vi "数据索引起始时间填补空白.vi"(8 "error in (no error)":errorcluster caption="错误输入（无错误）") -> (0 "error out":errorcluster caption="错误输出")   [LabVIEW 2016, in "数据传输系统.lvlib"]
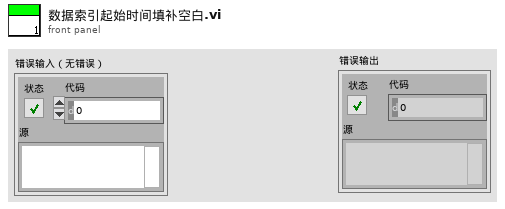
[diagram p1: front panel]
types:
  T1 = typedef "LVDateTimeRec.ctl" = cluster{"秒数的小数部分":dbl, "秒":i32, "分":i32, "时":i32, "日":i32, "月":i32, "年":i32, "天数（周）":i32, "天数（年）":i32, "DST":i32}
  T2 = cluster{"氨氮仪器参数索引起始时间":string, "总磷仪器参数索引起始时间":string, "总氮仪器参数索引起始时间":string, "CODMn仪器参数索引起始时间":string, "CODCr仪器参数索引起始时间":string, "DO仪器参数索引起始时间":string, "PH仪器参数索引起始时间":string, "比电导率仪器参数索引起始时间":string, "水温仪器参数索引起始时间":string, "浊度仪器参数索引起始时间":string, "叶绿素a仪器参数索引起始时间":string, "藻密度仪器参数索引起始时间":string, "ORP仪器参数索引起始时间":string}
  T3 = cluster{"氨氮加标回收索引起始时间":string, "总磷加标回收索引起始时间":string, "总氮加标回收索引起始时间":string, "CODMn加标回收索引起始时间":string, "CODCr加标回收索引起始时间":string}
  T4 = cluster{"氨氮标样核查索引起始时间":string, "总磷标样核查索引起始时间":string, "总氮标样核查索引起始时间":string, "CODMn标样核查索引起始时间":string, "CODCr标样核查索引起始时间":string, "DO标样核查索引起始时间":string, "PH标样核查索引起始时间":string, "比电导率标样核查索引起始时间":string, "水温标样核查索引起始时间":string, "浊度标样核查索引起始时间":string, "叶绿素a标样核查索引起始时间":string, "藻密度标样核查索引起始时间":string, "亚硝酸盐标样核查索引起始时间":string, "硫化物标样核查索引起始时间":string, "ORP标样核查索引起始时间":string}
  T5 = cluster{"氨氮跨度核查索引起始时间":string, "总磷跨度核查索引起始时间":string, "总氮跨度核查索引起始时间":string, "CODMn跨度核查索引起始时间":string, "CODCr跨度核查索引起始时间":string, "亚硝酸盐跨度核查索引起始时间":string, "硫化物跨度核查索引起始时间":string, "ORP跨度核查索引起始时间":string}
  T6 = cluster{"氨氮报警信息索引起始时间":string, "总磷报警信息索引起始时间":string, "总氮报警信息索引起始时间":string, "CODMn报警信息索引起始时间":string, "CODCr报警信息索引起始时间":string, "DO报警信息索引起始时间":string, "PH报警信息索引起始时间":string, "比电导率报警信息索引起始时间":string, "水温报警信息索引起始时间":string, "浊度报警信息索引起始时间":string, "叶绿素报警信息索引起始时间":string, "系统报警信息索引起始时间":string}
  T7 = cluster{"氨氮集成干预索引起始时间":string, "总磷集成干预索引起始时间":string, "总氮集成干预索引起始时间":string, "CODMn集成干预索引起始时间":string, "CODCr集成干预索引起始时间":string, "DO集成干预索引起始时间":string, "PH集成干预索引起始时间":string, "比电导率集成干预索引起始时间":string, "水温集成干预索引起始时间":string, "浊度集成干预索引起始时间":string, "叶绿素a集成干预索引起始时间":string, "藻密度集成干预索引起始时间":string, "亚硝酸盐集成干预索引起始时间":string, "硫化物集成干预索引起始时间":string, "ORP集成干预索引起始时间":string}
  T8 = cluster{"氨氮仪器日志索引起始时间":string, "总磷仪器日志索引起始时间":string, "总氮仪器日志索引起始时间":string, "CODMn仪器日志索引起始时间":string, "CODCr仪器日志索引起始时间":string, "系统仪器日志索引起始时间":string}
  T9 = cluster{"氨氮零点核查索引起始时间":string, "总磷零点核查索引起始时间":string, "总氮零点核查索引起始时间":string, "CODMn零点核查索引起始时间":string, "CODCr零点核查索引起始时间":string, "亚硝酸盐零点核查索引起始时间":string, "硫化物零点核查索引起始时间":string, "ORP零点核查索引起始时间":string}
  T10 = cluster{"氨氮平行样索引起始时间":string, "总磷平行样索引起始时间":string, "总氮平行样索引起始时间":string, "CODMn平行样索引起始时间":string, "CODCr平行样索引起始时间":string}
  T11 = cluster{"[0]":string, "[1]":string, "[2]":string, "[3]":string, "[4]":string, "[5]":string, "[6]":string, "[7]":string, "[8]":string, "[9]":string, "[10]":string, "[11]":string, "[12]":string}
  T12 = cluster{"[0]":string, "[1]":string, "[2]":string, "[3]":string, "[4]":string}
  T13 = cluster{"[0]":string, "[1]":string, "[2]":string, "[3]":string, "[4]":string, "[5]":string, "[6]":string, "[7]":string, "[8]":string, "[9]":string, "[10]":string, "[11]":string, "[12]":string, "[13]":string, "[14]":string}
  T14 = cluster{"[0]":string, "[1]":string, "[2]":string, "[3]":string, "[4]":string, "[5]":string, "[6]":string, "[7]":string}
  T15 = cluster{"[0]":string, "[1]":string, "[2]":string, "[3]":string, "[4]":string, "[5]":string, "[6]":string, "[7]":string, "[8]":string, "[9]":string, "[10]":string, "[11]":string}
  T16 = cluster{"[0]":string, "[1]":string, "[2]":string, "[3]":string, "[4]":string, "[5]":string}
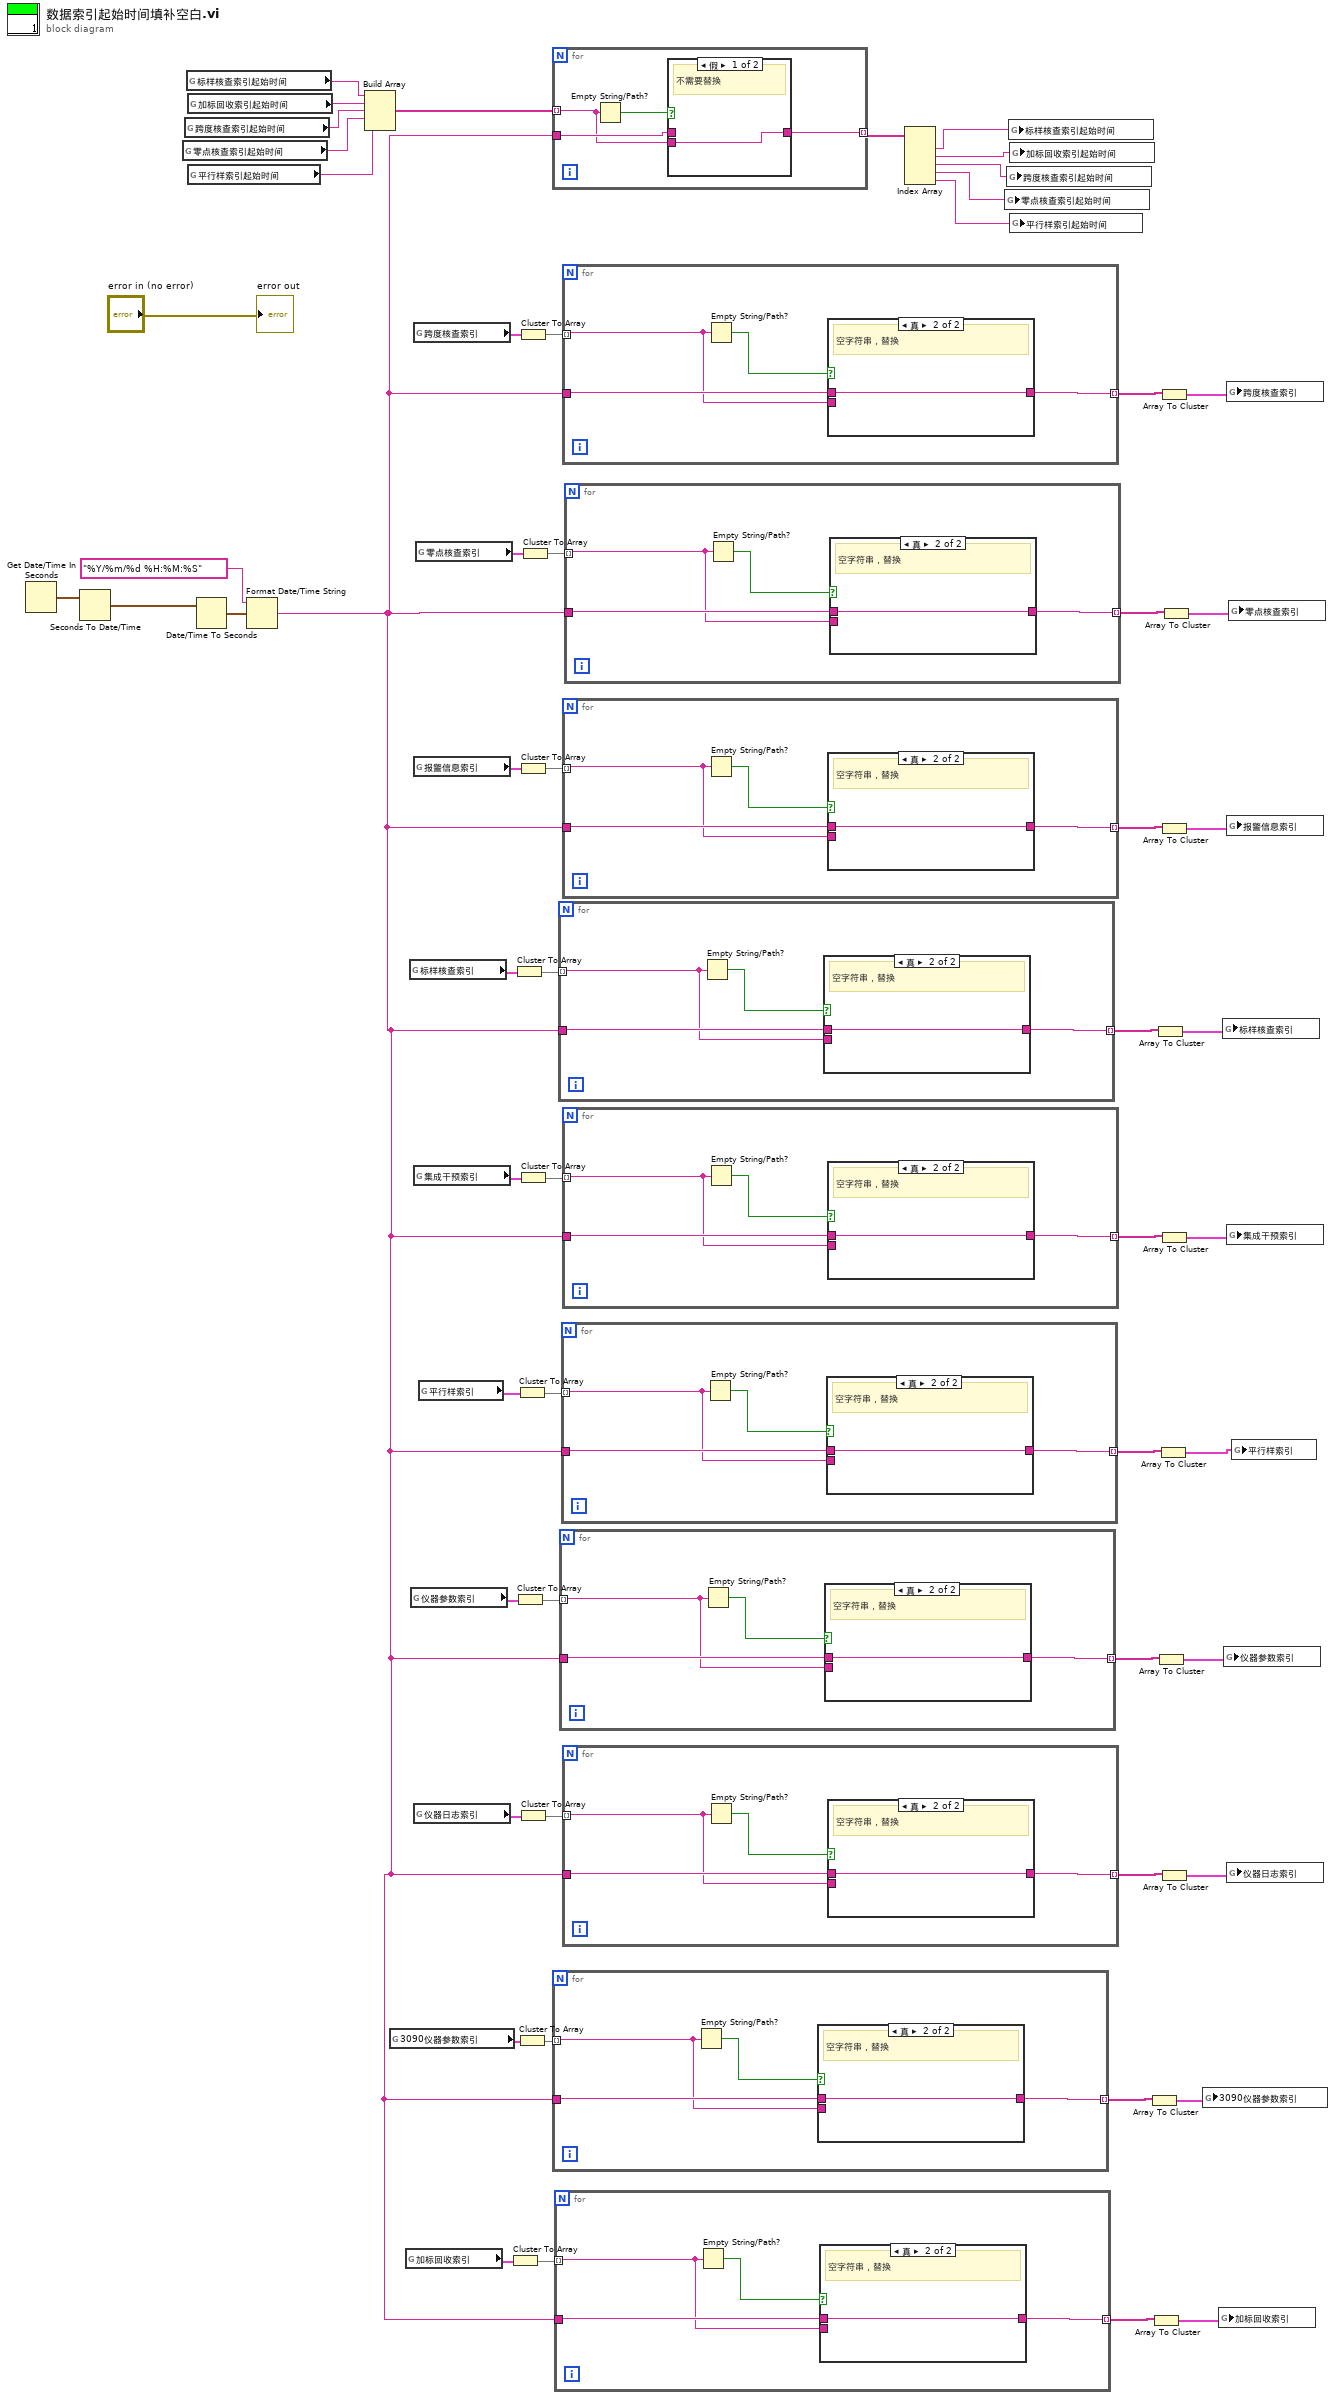
[diagram p0: block diagram]
diagram:
  n1 = Get Date/Time In Seconds() -> (seconds since 1Jan1904=w58:timestamp)
  n2 = Seconds To Date/Time(time stamp (now)=w58) -> (date time rec=w56:T1)  [unwired: 1 in]
  n3 = global read "全局 时间2.vi" "零点核查索引起始时间"() -> (w17:string)
  n4 = global read "全局 时间2.vi" "跨度核查索引起始时间"() -> (w19:string)
  n5 = global read "全局 时间2.vi" "标样核查索引起始时间"() -> (w21:string)
  n6 = global read "全局 时间2.vi" "加标回收索引起始时间"() -> (w20:string)
  n7 = global read "全局 时间2.vi" "平行样索引起始时间"() -> (w18:string)
  n8 = Date/Time To Seconds(2:w56) -> (0:w55:timestamp)  [unwired: 1 in]
  n9 = Format Date/Time String(time format string (%c)="%Y/%m/%d %H:%M:%S" ("时间格式字符串(%c)"), seconds (now)=w55) -> (date/time string=w1:string)  [unwired: 1 in]
  n10 = Build Array(w21, w20, w19, w17, w18) -> (w16:string[])
  n11 = global read "全局 时间2.vi" "3090仪器参数索引"() -> (w9:T2)
  n12 = global read "全局 时间2.vi" "加标回收索引"() -> (w5:T3)
  n13 = global read "全局 时间2.vi" "标样核查索引"() -> (w46:T4)
  n14 = global read "全局 时间2.vi" "仪器参数索引"() -> (w27:T2)
  n15 = global read "全局 时间2.vi" "跨度核查索引"() -> (w35:T5)
  n16 = global read "全局 时间2.vi" "报警信息索引"() -> (w47:T6)
  n17 = global read "全局 时间2.vi" "集成干预索引"() -> (w39:T7)
  n18 = global read "全局 时间2.vi" "仪器日志索引"() -> (w26:T8)
  n19 = global read "全局 时间2.vi" "零点核查索引"() -> (w54:T9)
  n20 = global read "全局 时间2.vi" "平行样索引"() -> (w34:T10)
  n21 = Cluster To Array(cluster=w5) -> (array=w4:string[])
  n22 = Cluster To Array(cluster=w46) -> (array=w45:string[])
  n23 = Cluster To Array(cluster=w27) -> (array=w28:string[])
  n24 = Cluster To Array(cluster=w34) -> (array=w33:string[])
  n25 = Cluster To Array(cluster=w9) -> (array=w8:string[])
  n26 = Cluster To Array(cluster=w35) -> (array=w36:string[])
  n27 = Cluster To Array(cluster=w47) -> (array=w48:string[])
  n28 = Cluster To Array(cluster=w39) -> (array=w40:string[])
  n29 = Cluster To Array(cluster=w26) -> (array=w25:string[])
  n30 = Cluster To Array(cluster=w54) -> (array=w53:string[])
  n31 = for {
    tunnel: w16 -> [w60] mode=indexing
    tunnel: w1 -> [w61]
    tunnel: [w59] -> w15 mode=indexing
    n32 = Empty String/Path?(string/path=w60) -> (empty?=w62:bool)
    n33 = case shown="假" w62 {
      tunnel: w61 -> [_ w64]
      tunnel: [w63 w64] -> w59
      tunnel: w60 -> [w63 _]
      frame False {
        # "不需要替换"
      }
      frame True {
        # "空字符串，替换"
      }
    }
  }
  n34 = for {
    tunnel: w8 -> [w65] mode=indexing
    tunnel: w1 -> [w67]
    tunnel: [w66] -> w7 mode=indexing
    n35 = Empty String/Path?(string/path=w65) -> (empty?=w68:bool)
    n36 = case shown="真" w68 {
      tunnel: w67 -> [_ w70]
      tunnel: [w69 w70] -> w66
      tunnel: w65 -> [w69 _]
      frame False {
        # "不需要替换"
      }
      frame True {
        # "空字符串，替换"
      }
    }
  }
  n37 = for {
    tunnel: w4 -> [w71] mode=indexing
    tunnel: w1 -> [w73]
    tunnel: [w72] -> w3 mode=indexing
    n38 = Empty String/Path?(string/path=w71) -> (empty?=w74:bool)
    n39 = case shown="真" w74 {
      tunnel: w73 -> [_ w76]
      tunnel: [w75 w76] -> w72
      tunnel: w71 -> [w75 _]
      frame False {
        # "不需要替换"
      }
      frame True {
        # "空字符串，替换"
      }
    }
  }
  n40 = for {
    tunnel: w45 -> [w77] mode=indexing
    tunnel: w1 -> [w79]
    tunnel: [w78] -> w44 mode=indexing
    n41 = Empty String/Path?(string/path=w77) -> (empty?=w80:bool)
    n42 = case shown="真" w80 {
      tunnel: w79 -> [_ w82]
      tunnel: [w81 w82] -> w78
      tunnel: w77 -> [w81 _]
      frame False {
        # "不需要替换"
      }
      frame True {
        # "空字符串，替换"
      }
    }
  }
  n43 = for {
    tunnel: w28 -> [w83] mode=indexing
    tunnel: w1 -> [w85]
    tunnel: [w84] -> w29 mode=indexing
    n44 = Empty String/Path?(string/path=w83) -> (empty?=w86:bool)
    n45 = case shown="真" w86 {
      tunnel: w85 -> [_ w88]
      tunnel: [w87 w88] -> w84
      tunnel: w83 -> [w87 _]
      frame False {
        # "不需要替换"
      }
      frame True {
        # "空字符串，替换"
      }
    }
  }
  n46 = for {
    tunnel: w33 -> [w89] mode=indexing
    tunnel: w1 -> [w91]
    tunnel: [w90] -> w32 mode=indexing
    n47 = Empty String/Path?(string/path=w89) -> (empty?=w92:bool)
    n48 = case shown="真" w92 {
      tunnel: w91 -> [_ w94]
      tunnel: [w93 w94] -> w90
      tunnel: w89 -> [w93 _]
      frame False {
        # "不需要替换"
      }
      frame True {
        # "空字符串，替换"
      }
    }
  }
  n49 = for {
    tunnel: w36 -> [w95] mode=indexing
    tunnel: w1 -> [w97]
    tunnel: [w96] -> w37 mode=indexing
    n50 = Empty String/Path?(string/path=w95) -> (empty?=w98:bool)
    n51 = case shown="真" w98 {
      tunnel: w97 -> [_ w100]
      tunnel: [w99 w100] -> w96
      tunnel: w95 -> [w99 _]
      frame False {
        # "不需要替换"
      }
      frame True {
        # "空字符串，替换"
      }
    }
  }
  n52 = for {
    tunnel: w48 -> [w101] mode=indexing
    tunnel: w1 -> [w103]
    tunnel: [w102] -> w49 mode=indexing
    n53 = Empty String/Path?(string/path=w101) -> (empty?=w104:bool)
    n54 = case shown="真" w104 {
      tunnel: w103 -> [_ w106]
      tunnel: [w105 w106] -> w102
      tunnel: w101 -> [w105 _]
      frame False {
        # "不需要替换"
      }
      frame True {
        # "空字符串，替换"
      }
    }
  }
  n55 = for {
    tunnel: w40 -> [w107] mode=indexing
    tunnel: w1 -> [w109]
    tunnel: [w108] -> w41 mode=indexing
    n56 = Empty String/Path?(string/path=w107) -> (empty?=w110:bool)
    n57 = case shown="真" w110 {
      tunnel: w109 -> [_ w112]
      tunnel: [w111 w112] -> w108
      tunnel: w107 -> [w111 _]
      frame False {
        # "不需要替换"
      }
      frame True {
        # "空字符串，替换"
      }
    }
  }
  n58 = for {
    tunnel: w25 -> [w113] mode=indexing
    tunnel: w1 -> [w115]
    tunnel: [w114] -> w24 mode=indexing
    n59 = Empty String/Path?(string/path=w113) -> (empty?=w116:bool)
    n60 = case shown="真" w116 {
      tunnel: w115 -> [_ w118]
      tunnel: [w117 w118] -> w114
      tunnel: w113 -> [w117 _]
      frame False {
        # "不需要替换"
      }
      frame True {
        # "空字符串，替换"
      }
    }
  }
  n61 = for {
    tunnel: w53 -> [w119] mode=indexing
    tunnel: w1 -> [w121]
    tunnel: [w120] -> w52 mode=indexing
    n62 = Empty String/Path?(string/path=w119) -> (empty?=w122:bool)
    n63 = case shown="真" w122 {
      tunnel: w121 -> [_ w124]
      tunnel: [w123 w124] -> w120
      tunnel: w119 -> [w123 _]
      frame False {
        # "不需要替换"
      }
      frame True {
        # "空字符串，替换"
      }
    }
  }
  n64 = Index Array(array=w15) -> (element #1=w14:string, element #2=w13:string, element #3=w12:string, element #4=w10:string, element #5=w11:string)  [unwired: 5 in]
  n65 = global write "全局 时间2.vi" "零点核查索引起始时间"(w10) -> ()
  n66 = global write "全局 时间2.vi" "跨度核查索引起始时间"(w12) -> ()
  n67 = global write "全局 时间2.vi" "标样核查索引起始时间"(w14) -> ()
  n68 = global write "全局 时间2.vi" "加标回收索引起始时间"(w13) -> ()
  n69 = global write "全局 时间2.vi" "平行样索引起始时间"(w11) -> ()
  n70 = Array To Cluster(array=w7) -> (cluster=w6:T11)
  n71 = Array To Cluster(array=w3) -> (cluster=w2:T12)
  n72 = Array To Cluster(array=w44) -> (cluster=w43:T13)
  n73 = Array To Cluster(array=w29) -> (cluster=w30:T11)
  n74 = Array To Cluster(array=w32) -> (cluster=w31:T12)
  n75 = Array To Cluster(array=w37) -> (cluster=w38:T14)
  n76 = Array To Cluster(array=w49) -> (cluster=w50:T15)
  n77 = Array To Cluster(array=w41) -> (cluster=w42:T13)
  n78 = Array To Cluster(array=w24) -> (cluster=w23:T16)
  n79 = Array To Cluster(array=w52) -> (cluster=w51:T14)
  n80 = global write "全局 时间2.vi" "3090仪器参数索引"(w6) -> ()
  n81 = global write "全局 时间2.vi" "加标回收索引"(w2) -> ()
  n82 = global write "全局 时间2.vi" "标样核查索引"(w43) -> ()
  n83 = global write "全局 时间2.vi" "仪器参数索引"(w30) -> ()
  n84 = global write "全局 时间2.vi" "跨度核查索引"(w38) -> ()
  n85 = global write "全局 时间2.vi" "报警信息索引"(w50) -> ()
  n86 = global write "全局 时间2.vi" "集成干预索引"(w42) -> ()
  n87 = global write "全局 时间2.vi" "仪器日志索引"(w23) -> ()
  n88 = global write "全局 时间2.vi" "零点核查索引"(w51) -> ()
  n89 = global write "全局 时间2.vi" "平行样索引"(w31) -> ()
  "error out" <- "error in (no error)"
